vi "Local Variables.vi"() -> ()   [LabVIEW 2019]
doc: "This VI creates two queues to pass data between parallel loops. Queues are most useful when you need to send data from one or more data sources to one data sink with no potential loss of data."
panel:
  in  "Receiving Loop timing":u32=500
  out "Received Data":dbl(graph)
  out "Generated Data":dbl(graph)
  in  "Stop":bool
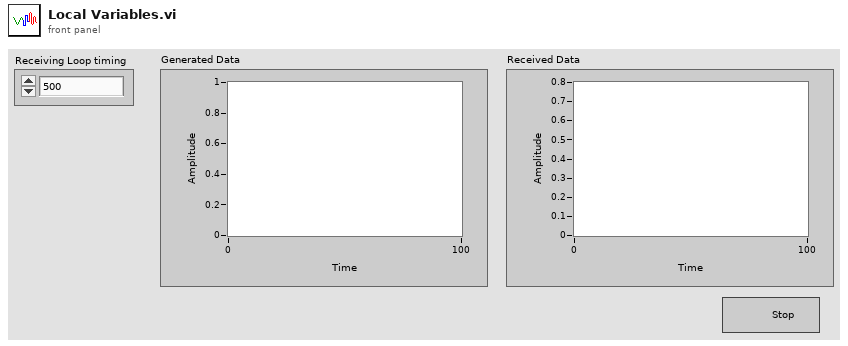
[diagram p1: front panel]
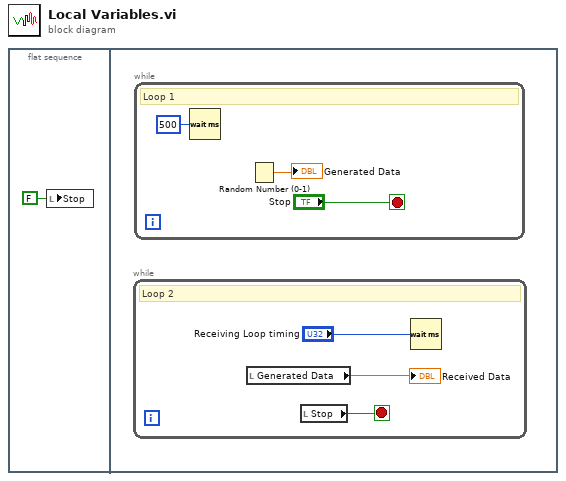
[diagram p0: block diagram]
diagram:
  n1 = flat-sequence {
    frame #0 {
      n2 = local write "Stop"(FALSE ("Stop")) -> ()
    }
    frame #1 {
      n3 = while {
        stop <- w4 stop-if-true
        # "Loop 2"
        n4 = local read "Generated Data"() -> (→"Received Data":dbl)
        n5 = local read "Stop"() -> (w4:bool)
        n6 = Wait (ms)(milliseconds to wait="Receiving Loop timing") -> ()  [unwired: 1 out]
      }
      n7 = while {
        stop <- "Stop" stop-if-true
        # "Loop 1"
        n8 = Wait (ms)(milliseconds to wait=u32 500) -> ()  [unwired: 1 out]
        n9 = Random Number (0-1)() -> (number: 0 to 1=→"Generated Data":dbl)
      }
    }
  }
